vi "addBSONElementt.vi"(6 "Add to front of object (false)":bool, 8 "error in (no error)":errorcluster, 9 "Element":refnum<class "tBSONElement.lvclass">, 10 "Replace? (false)":bool, 11 "tBSONDocument in":refnum<class "tBSONDocument.lvclass">) -> (0 "error out":errorcluster, 3 "tBSONDocument out":refnum<class "tBSONDocument.lvclass">)   [LabVIEW 2013, in "BSON.lvlib" / "tBSONDocument.lvclass"]
doc: "Adds a BSON Element to a BSON document."
uses:
  tBSONDocument.lvclass
  tBSONElement/tBSONElement.lvclass
  tBSONDocument.lvclass/tBSONDocument.ctl
  tBSONElement/getName.vi
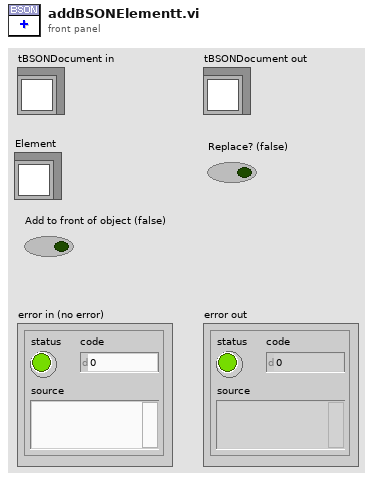
[diagram p1: front panel]
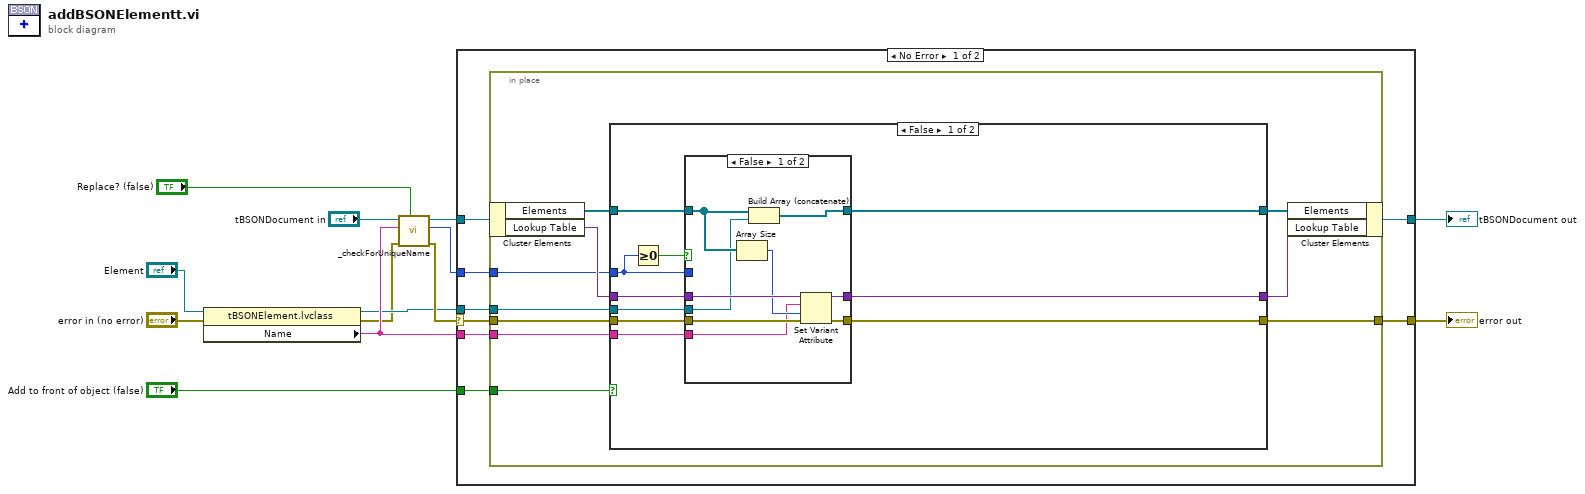
[diagram p0: block diagram]
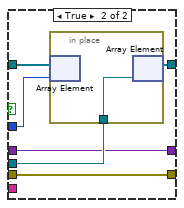
[diagram p2: hidden frame]
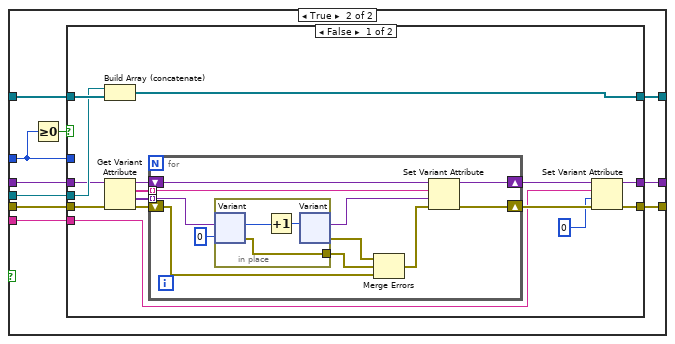
[diagram p3: hidden frame]
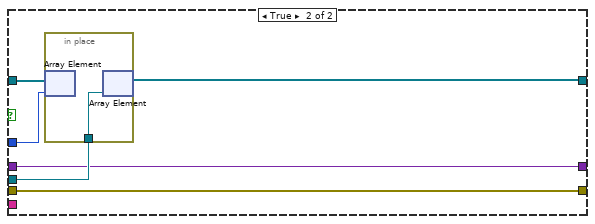
[diagram p4: hidden frame]
diagram:
  n1 = property class="tBSONElement.lvclass"(reference="Element", error in="error in (no error)") -> (reference out=w5:refnum<class "tBSONElement.lvclass">, error out=w4:errorcluster, "Name"=w6:string)
  n2 = call "_checkForUniqueName.vi"("Replace?"="Replace? (false)", "error in (no error)"=w4, "Name"=w6, "tBSONDocument in"="tBSONDocument in") -> ("error out"=w10:errorcluster, "Replace Index"=w2:i32, "tBSONDocument out"=w11:refnum<class "tBSONDocument.lvclass">)  [unwired: 5 in]
  n3 = case shown="No Error" w10 {
    selector: w10 -> [w18 w105]
    tunnel: [w21 w105] -> w13
    tunnel: [w20 w104] -> w12
    tunnel: w11 -> [w19 w104]
    tunnel: w6 -> [w17 _]
    tunnel: w5 -> [w16 _]
    tunnel: "Add to front of object (false)" -> [w15 _]
    tunnel: w2 -> [w14 _]
    frame No Error {
      n4 = in-place {
        in-place-border: [w30] -> w21
        in-place-border: w18 -> [w26]
        in-place-border: w17 -> [w25]
        in-place-border: w16 -> [w24]
        in-place-border: w15 -> [w23]
        in-place-border: w14 -> [w22]
        n5 = in-place-cluster #1(w19) -> ("Elements"=w27:refnum<class "tBSONElement.lvclass">[], "Lookup Table"=w31:variant)
        n6 = case shown="False" w23 {
          tunnel: w31 -> [w41 w64]
          tunnel: [w40 w61] -> w30
          tunnel: [w39 w62] -> w29
          tunnel: [w38 w65] -> w28
          tunnel: w27 -> [w37 w67]
          tunnel: w26 -> [w36 w63]
          tunnel: w25 -> [w35 w60]
          tunnel: w24 -> [w34 w66]
          tunnel: w22 -> [w32 w58]
          frame False {
            n7 = Greater Or Equal To 0?(x=w32) -> (x >= 0?=w33:bool)
            n8 = case shown="False" w33 {
              tunnel: w41 -> [w50 w52]
              tunnel: [w49 w51] -> w40
              tunnel: [w48 w52] -> w39
              tunnel: [w47 w53] -> w38
              tunnel: w37 -> [w46 w56]
              tunnel: w36 -> [w44 w51]
              tunnel: w35 -> [w43 _]
              tunnel: w34 -> [w42 w54]
              tunnel: w32 -> [_ w55]
              frame False {
                n9 = Array Size(array=w46) -> (size(s)=w45:i32)
                n10 = Build Array (concatenate)(w46, w42) -> (w47:refnum<class "tBSONElement.lvclass">[])
                n11 = Set Variant Attribute(Variant=w50, name=w43, value=w45, error in=w44) -> (Variant out=w48:variant, error out=w49:errorcluster)  [unwired: 1 out]
              }
              frame True {
                n12 = in-place {
                  in-place-border: w54 -> [w57]
                  n13 = in-place-array #2(w56, w55) -> ()  [unwired: 1 out]
                  n14 = in-place-array #2(w57) -> (w53:refnum<class "tBSONElement.lvclass">[])  [unwired: 1 out]
                }
              }
            }
          }
          frame True {
            n15 = Greater Or Equal To 0?(x=w58) -> (x >= 0?=w59:bool)
            n16 = case shown="False" w59 {
              tunnel: w67 -> [w82 w102]
              tunnel: w66 -> [w81 w100]
              tunnel: [w80 w99] -> w65
              tunnel: w64 -> [w79 w97]
              tunnel: w63 -> [w78 w98]
              tunnel: [w71 w97] -> w62
              tunnel: [w70 w98] -> w61
              tunnel: w60 -> [w69 _]
              tunnel: w58 -> [_ w101]
              frame False {
                n17 = Build Array (concatenate)(w81, w82) -> (w80:refnum<class "tBSONElement.lvclass">[])
                n18 = Get Variant Attribute(Variant=w79, error in=w78) -> (duplicate Variant=w77:variant, names=w76:string[], values=w75:variant[], error out=w74:errorcluster)  [unwired: 2 in]
                n19 = for {
                  tunnel: w76 -> [w90] mode=indexing
                  tunnel: w75 -> [w89] mode=indexing
                  shift-right: [w92] -> w73
                  shift-left: w77 -> [w91]
                  shift-right: [w93] -> w72
                  shift-left: w74 -> [w85]
                  n20 = in-place {
                    in-place-border: [w94] -> w86
                    n21 = in-place-variant #3(w89, 0) -> (w96:i32, w94:errorcluster)
                    n22 = Increment(x=w96) -> (x+1=w95:i32)
                    n23 = in-place-variant #3(w95) -> (w83:variant, w87:errorcluster)
                  }
                  n24 = Merge Errors(w87, w86, w85) -> (w84:errorcluster)
                  n25 = Set Variant Attribute(Variant=w91, name=w90, value=w83, error in=w84) -> (Variant out=w92:variant, error out=w93:errorcluster)  [unwired: 1 out]
                }
                n26 = Set Variant Attribute(Variant=w73, name=w69, value=0, error in=w72) -> (Variant out=w71:variant, error out=w70:errorcluster)  [unwired: 1 out]
              }
              frame True {
                n27 = in-place {
                  in-place-border: w100 -> [w103]
                  n28 = in-place-array #4(w102, w101) -> ()  [unwired: 1 out]
                  n29 = in-place-array #4(w103) -> (w99:refnum<class "tBSONElement.lvclass">[])  [unwired: 1 out]
                }
              }
            }
          }
        }
        n30 = in-place-cluster #1("Elements"=w28, "Lookup Table"=w29) -> (w20:refnum<class "tBSONDocument.lvclass">)
      }
    }
    frame Error {
    }
  }
  "error out" <- w13
  "tBSONDocument out" <- w12
